vi "FileWrite.vi"(4 "DataArray":dbl[](array[numeric]), 6 "FileFormat":string[](array[string]), 7 "Delimeter":string=",", 8 "Error In":errorcluster, 9 "Time Stamp":timestamp, 10 "Index":i32, 11 "refnum in":refnum<file>) -> (0 "Error Out":errorcluster, 3 "Byte Stream File Refnum":refnum<file>)   [LabVIEW 2017]
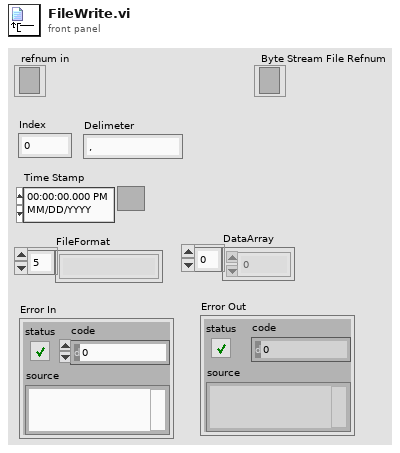
[diagram p1: front panel]
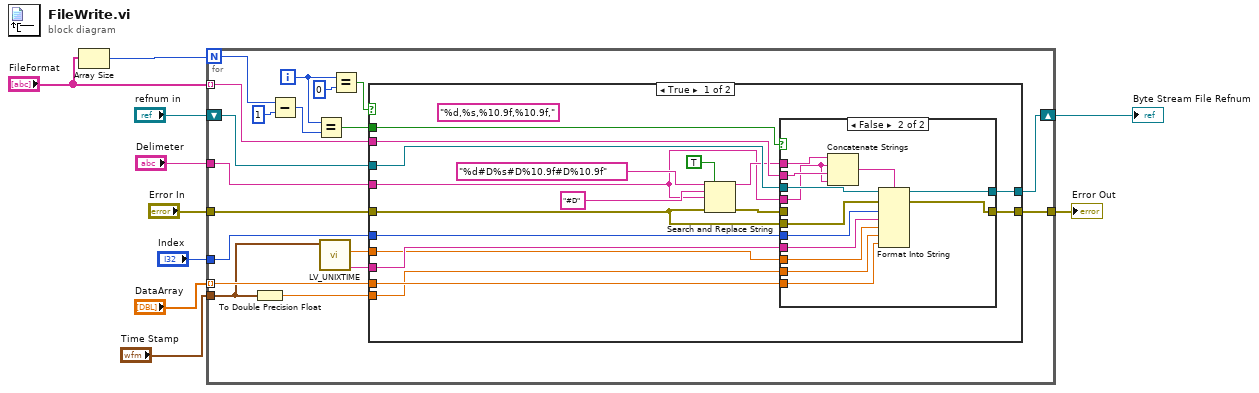
[diagram p0: block diagram]
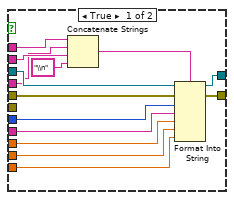
[diagram p2: hidden frame]
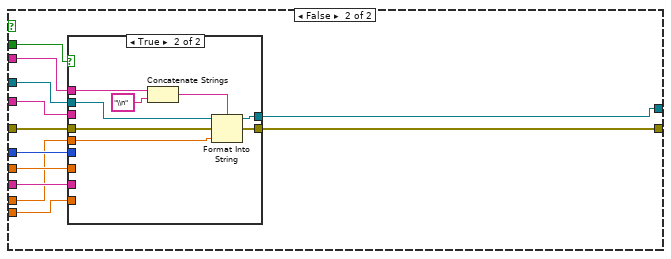
[diagram p3: hidden frame]
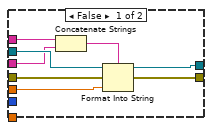
[diagram p4: hidden frame]
diagram:
  n1 = Array Size(array="FileFormat") -> (size(s)=w10:i32)
  n2 = for {
    N: w10 -> [w22]
    tunnel: [w25] -> w8
    tunnel: "Error In" -> [w23]
    shift-right: [w24] -> w9
    shift-left: "refnum in" -> [w19]
    tunnel: "Time Stamp" -> [w13]
    tunnel: "Index" -> [w18]
    tunnel: "DataArray" -> [w15] mode=indexing
    tunnel: "FileFormat" -> [w14] mode=indexing
    tunnel: "Delimeter" -> [w11]
    i -> [w27]
    n3 = To Double Precision Float(number=w13) -> (double precision float=w12:dbl)
    n4 = Subtract(x=w22, y=1 ("x")) -> (x-y=w21:i32)
    n5 = Equal?(x=w27, y=w21) -> (x = y?=w26:bool)
    n6 = call "LV_UNIXTIME.vi"("current time"=w13) -> ("date/time string"=w17:string, "UNIX time (s)"=w16:dbl)  [unwired: 9 in]
    n7 = Equal?(x=w27, y=0) -> (x = y?=w28:bool)
    n8 = case shown="True" w28 {
      tunnel: w19 -> [w46 w85]
      tunnel: w26 -> [w45 w84]
      tunnel: [w43 w82] -> w25
      tunnel: [w44 w83] -> w24
      tunnel: w23 -> [w42 w81]
      tunnel: w18 -> [w41 w80]
      tunnel: w17 -> [w40 w79]
      tunnel: w16 -> [w39 w78]
      tunnel: w15 -> [w38 w77]
      tunnel: w14 -> [w37 w76]
      tunnel: w12 -> [w36 w75]
      tunnel: w11 -> [w31 w74]
      frame True {
        (unwired) "%d,%s,%10.9f,%10.9f," ("format string")
        n9 = Search and Replace String(replace all?=TRUE ("ignore case? (F)"), input string="%d#D%s#D%10.9f#D%10.9f" ("format string"), search string="#D" ("format string"), replace string=w31, error in=w42) -> (result string=w33:string, error out=w32:errorcluster)  [unwired: 3 in, 2 out]
        n10 = case shown="False" w45 {
          tunnel: w46 -> [w60 w73]
          tunnel: [w59 w72] -> w44
          tunnel: [w58 w71] -> w43
          tunnel: w42 -> [_ w70]
          tunnel: w41 -> [w57 w69]
          tunnel: w40 -> [w56 w68]
          tunnel: w39 -> [w55 w67]
          tunnel: w38 -> [w54 w66]
          tunnel: w37 -> [w52 w62]
          tunnel: w36 -> [w50 w64]
          tunnel: w33 -> [w48 w63]
          tunnel: w32 -> [w49 _]
          tunnel: w31 -> [w47 w61]
          frame True {
            n11 = Concatenate Strings(w48, w47, w52, "\\n" ("string")) -> (w53:string)
            n12 = Format Into String(format string=w53, initial string=w60, error in=w49, w57, w56, w55, w50, w54) -> (resulting string=w59:refnum<file>, error out=w58:errorcluster)
          }
          frame False {
            n13 = Concatenate Strings(w63, w61, w62, w61) -> (w65:string)
            n14 = Format Into String(format string=w65, initial string=w73, error in=w70, w69, w68, w67, w64, w66) -> (resulting string=w72:refnum<file>, error out=w71:errorcluster)
          }
        }
      }
      frame False {
        n15 = case shown="True" w84 {
          tunnel: w85 -> [w93 w101]
          tunnel: [w92 w100] -> w83
          tunnel: [w91 w99] -> w82
          tunnel: w81 -> [w90 w98]
          tunnel: w80 -> [_ _]
          tunnel: w79 -> [_ _]
          tunnel: w78 -> [_ _]
          tunnel: w77 -> [w89 w97]
          tunnel: w76 -> [w88 w96]
          tunnel: w75 -> [_ _]
          tunnel: w74 -> [w86 _]
          frame False {
            n16 = Concatenate Strings(w88, w86) -> (w87:string)
            n17 = Format Into String(format string=w87, initial string=w93, error in=w90, w89) -> (resulting string=w92:refnum<file>, error out=w91:errorcluster)
          }
          frame True {
            n18 = Concatenate Strings(w96, "\\n" ("string")) -> (w95:string)
            n19 = Format Into String(format string=w95, initial string=w101, error in=w98, w97) -> (resulting string=w100:refnum<file>, error out=w99:errorcluster)
          }
        }
      }
    }
  }
  "Byte Stream File Refnum" <- w9
  "Error Out" <- w8
